vi "Configure ARB Sequence CDWell Level.vi"(7 "Level2(0)  2":dbl, 8 "error in (no error)":errorcluster, 9 "Level(0)":dbl, 10 "Step(1)":i32=1, 11 "VISA resource name":refnum<visa-resource-name>) -> (0 "error out":errorcluster, 3 "VISA resource name out":refnum<visa-resource-name>)   [LabVIEW 2015, in "IT6000C.lvlib"]
doc: "This command is used to set the Sequence of the currently selected step N CDWell waveform in a step (or points) of high and low amplitude, which specifies a point level, specify a value for the unit with the amp or volts, minimum and maximum values taken in equipment rating this command contains three parameters, the first < + > the NRf said high amplitude, the second < + > the NRf said low amplitude, the third parameter < NR1 > says the specified steps (or points), and the first parameter value must be greater than the second parameter Settings."
uses:
  <instrlib>/IT6000C/IT6000C.lvlib
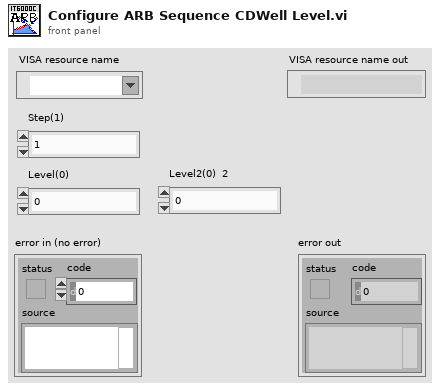
[diagram p1: front panel]
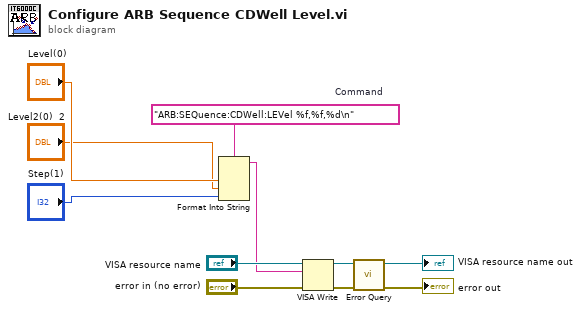
[diagram p0: block diagram]
diagram:
  w5 = "ARB:SEQuence:CDWell:LEVel %f,%f,%d\n"  # Command
  n1 = Format Into String(format string=w5, "Level(0)", "Level2(0)  2", "Step(1)") -> (resulting string=w4:string)  [unwired: 2 in, 1 out]
  n2 = VISA Write(VISA resource name="VISA resource name", write buffer=w4, error in (no error)="error in (no error)") -> (VISA resource name out=w8:refnum<visa-resource-name>, error out=w9:errorcluster)  [unwired: 1 out]
  n3 = call <instrlib>:"Error Query.vi"("error in (no error)"=w9, "VISA resource name"=w8) -> ("error out"=→"error out":errorcluster, "VISA resource name out"=→"VISA resource name out":refnum<visa-resource-name>)  [unwired: 6 in, 2 out]
